vi "test_Delete Instrument Addon_Check correct Instrument Addon remains after deletion.vi"(8 "error in (no error)":errorcluster, 11 "TestCase in":refnum<class "Instrument Addon Scripting API Custom Device Unit Tests.lvclass">) -> (0 "error out":errorcluster, 3 "TestCase out":refnum<class "Instrument Addon Scripting API Custom Device Unit Tests.lvclass">)   [LabVIEW 2018, in "Instrument Addon Scripting API Custom Device Unit Tests.lvclass"]
uses:
  Instrument Addon Scripting API Custom Device Unit Tests.lvclass
  NationalInstruments.VeriStand.SystemDefinitionAPI
  Addon/Addon Shared/SubVIs/Constants.vi
  <vilib>/addons/_JKI Toolkits/VI Tester/TestCase.llb/TestCase.lvclass
  Instrument Addon Scripting API Test Assets/Instrument Addon Scripting API Test Assets.lvclass
  APIs/Scripting API/Instrument Addon Scripting API.lvlib
  Addon/Addon Shared/Instrument Addon Shared.lvlib
  C:/Program Files (x86)/National Instruments/LabVIEW 2018/vi.lib/addons/_JKI Toolkits/VI Tester/TestCase.llb/TestCase.lvclass
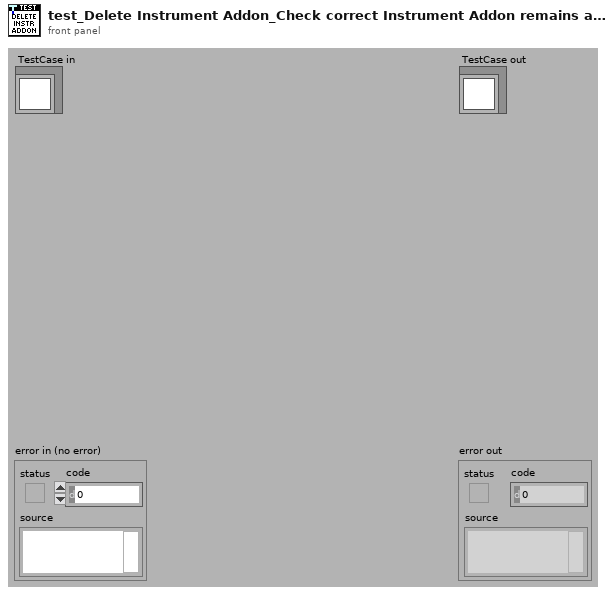
[diagram p1: front panel]
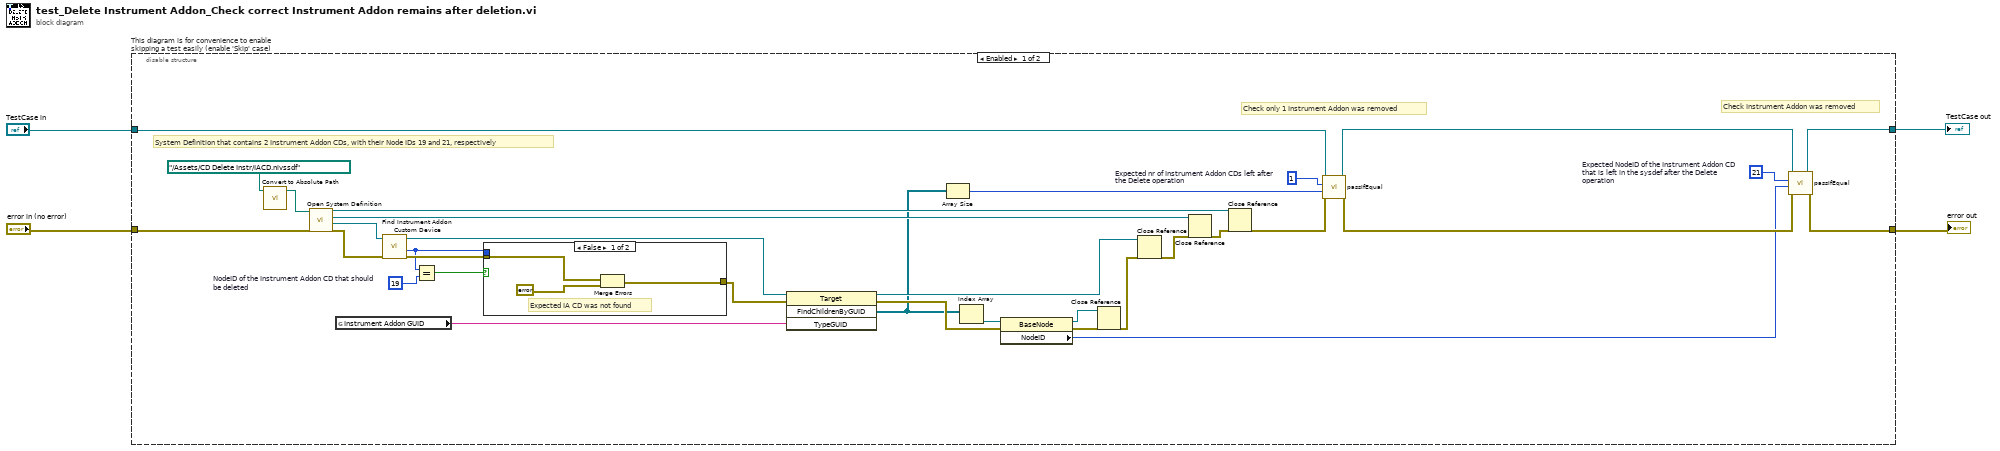
[diagram p0: block diagram]
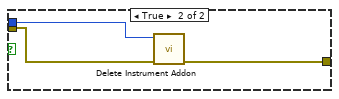
[diagram p2: hidden frame]
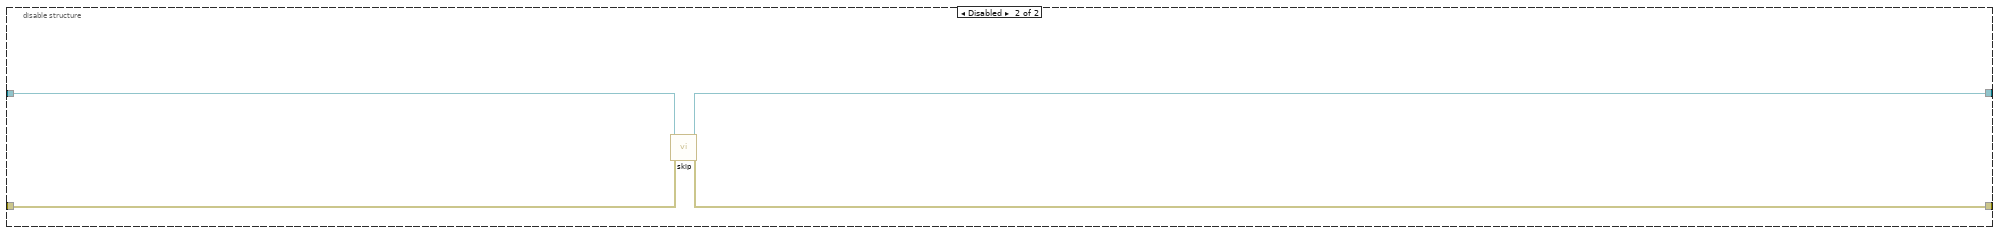
[diagram p3: hidden frame]
diagram:
  n1 = disable-structure "This diagram is for convenience to enable skipping a test easily (enable 'Skip' case)" shown="Enabled" {
    disable-tunnel: "TestCase in" -> [w7 w45]
    disable-tunnel: [w32 w44] -> w1
    disable-tunnel: [w33 w47] -> w3
    disable-tunnel: "error in (no error)" -> [w37 w46]
    frame Enabled {
      w8 = 1  # Expected nr of Instrument Addon CDs left after the Delete operation
      w13 = u64 21  # Expected NodeID of the Instrument Addon CD that is left in the sysdef after the Delete operation
      w23 = u64 19  # NodeID of the Instrument Addon CD that should be deleted
      # "Check only 1 Instrument Addon was removed"
      # "System Definition that contains 2 Instrument Addon CDs, with their Node IDs 19 and 21, respectively"
      # "Check Instrument Addon was removed"
      n2 = call "Convert to Absolute Path.vi"("System Definition File"=path "../Assets/CD Delete Instr/IACD.nivssdf" ("SDF file")) -> ("Absolute Path"=w36:path)  [unwired: 10 in]
      n3 = call "Open System Definition.vi"("error in (no error)"=w37, "System Definition File"=w36) -> ("error out"=w31:errorcluster, "Target Refnum"=w21:refnum<k24>, "Root Refnum"=w35:refnum<k24>, "System Definition Refnum"=w34:refnum<k24>)  [unwired: 6 in]
      n4 = global read "Constants.vi" "Instrument Addon GUID"() -> (w20:string)
      n5 = call "Find Instrument Addon Custom Device.vi"("error in"=w31, "target in"=w21) -> ("error out"=w30:errorcluster, "NodeID"=w24:u64, "target out"=w27:refnum<k24>)  [unwired: 7 in]
      n6 = Equal?(x=w24, y=w23) -> (x = y?=w22:bool)
      n7 = case shown="False" w22 {
        tunnel: w30 -> [w40 w43]
        tunnel: [w38 w42] -> w29
        tunnel: w24 -> [_ w41]
        frame False {
          # "Expected IA CD was not found"
          n8 = Merge Errors(w40, errorcluster {"status"=TRUE, "code"=0, "source"="Sysdef does not contain a Instrument Addon Custom Device"} ("error out")) -> (w38:errorcluster)
        }
        frame True {
          n9 = call "Delete Instrument Addon.vi"("error in (no error)"=w43, "Instrument Addon Refnum"=w41) -> ("error out"=w42:errorcluster)  [unwired: 9 in]
        }
      }
      n10 = invoke class="Target" method="FindChildrenByGUID"(reference=w27, error in=w29, "TypeGUID"=w20) -> (reference out=w17:refnum<k24>, error out=w18:errorcluster, "FindChildrenByGUID"=w12:refnum<k24>[])  [unwired: 1 in, 1 out]
      n11 = Array Size(array=w12) -> (size(s)=w9:i32)
      n12 = Index Array(array=w12) -> (element=w19:refnum<k24>)  [unwired: 1 in]
      n13 = property class="BaseNode"(reference=w19, error in=w18) -> (reference out=w15:refnum<k24>, error out=w16:errorcluster, "NodeID"=w5:u64)
      n14 = Close Reference(reference=w15, error in (no error)=w16) -> (error out=w14:errorcluster)
      n15 = Close Reference(reference=w17, error in (no error)=w14) -> (error out=w26:errorcluster)
      n16 = Close Reference(reference=w35, error in (no error)=w26) -> (error out=w25:errorcluster)
      n17 = Close Reference(reference=w34, error in (no error)=w25) -> (error out=w11:errorcluster)
      n18 = call-dynamic "passIfEqual.vi"("error in (no error)"=w11, "y"=w9, "x"=w8, "TestCase in"=w7) -> ("error out"=w10:errorcluster, "TestCase out"=w6:refnum<class "Instrument Addon Scripting API Custom Device Unit Tests.lvclass">)  [unwired: 6 in]
      n19 = call-dynamic "passIfEqual.vi"("error in (no error)"=w10, "y"=w5, "x"=w13, "TestCase in"=w6) -> ("error out"=w33:errorcluster, "TestCase out"=w32:refnum<class "Instrument Addon Scripting API Custom Device Unit Tests.lvclass">)  [unwired: 6 in]
    }
    frame Disabled {
      # "skip test result while test is under development"
      n20 = call <vilib>:"skip.vi"("error in (no error)"=w46, "TestCase in"=w45) -> ("error out"=w47:errorcluster, "TestCase out"=w44:refnum<class "Instrument Addon Scripting API Custom Device Unit Tests.lvclass">)  [unwired: 8 in]
    }
  }
  "error out" <- w3
  "TestCase out" <- w1
